vi "3.4.vi"(2 "字符串 3":string, 3 "字符串 2":string, 4 "字符串":string) -> (0 "长度":i32, 1 "结果字符串":string)   [LabVIEW 2017]
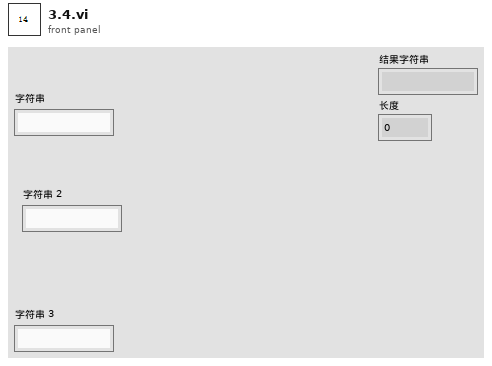
[diagram p1: front panel]
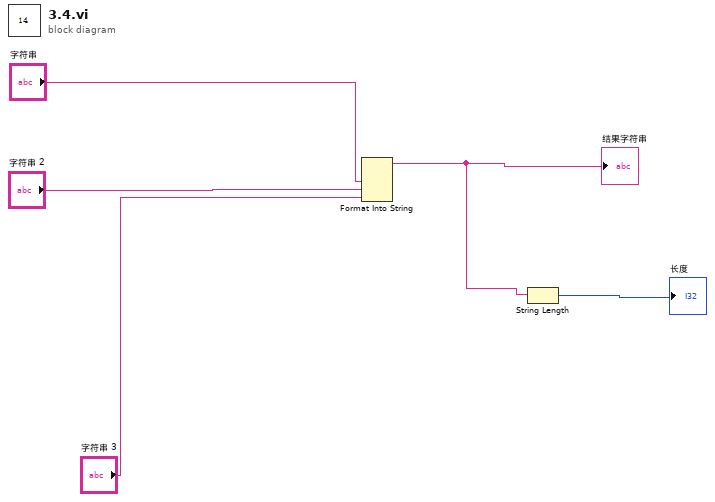
[diagram p0: block diagram]
diagram:
  n1 = Format Into String("字符串", "字符串 2", "字符串 3") -> (resulting string=w2:string)  [unwired: 3 in, 1 out]
  "结果字符串" <- w2
  n2 = String Length(string=w2) -> (length=→"长度":i32)
